vi "Menu Handler.vi"(8 "error in (no error)":errorcluster, 9 "ItemTag":string, 10 "Menu in":refnum<k9>, 11 "queue in":refnum<queue>) -> (0 "Error Out":errorcluster, 3 "Log 10?":bool=TRUE)   [LabVIEW 2014]
uses:
  Type Defs/OCT Hardware States.ctl
  DAQ Status States.ctl
  Classes/DAQ Control Functional Global States.ctl
  Classes/Processing/View A-Scan.vi
  Classes/Processing.lvclass
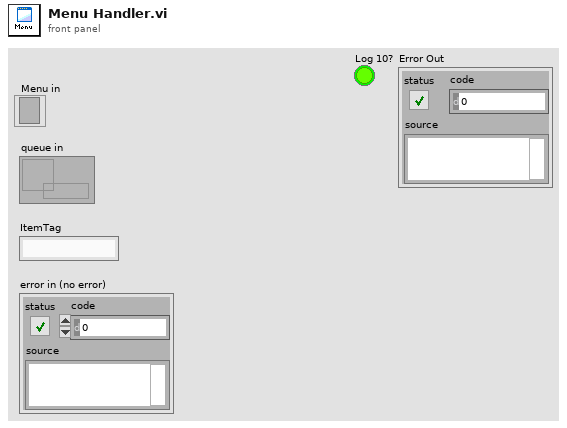
[diagram p1: front panel]
types:
  T1 = enum32{"Invalid", "Standard", "Closed", "Hidden", "Minimized", "Maximized"}
  T2 = typedef "DAQ Status States.ctl" = enum16{"Get", "Show"}
  T3 = typedef "OCT Hardware States.ctl" = enum16{"Acquire Data", "Initialize Laser", "Initialize Galvos", "Startup", "Reset DAQ", "Background Subtraction", "Acquire Background", "Update DAQ Parameters", "Stop", "Set Clock", "Initialize DAQ", "Set Resampling Array", "Save Sweep", "Configure Laser", "128 x 128", "512 x 1", "512 x 512", "Review Data"}
  T4 = typedef "DAQ Control Functional Global States.ctl" = enum16{"Status", "Set Processing Finished", "Reset", "Clear", "Set DAQ Finished"}
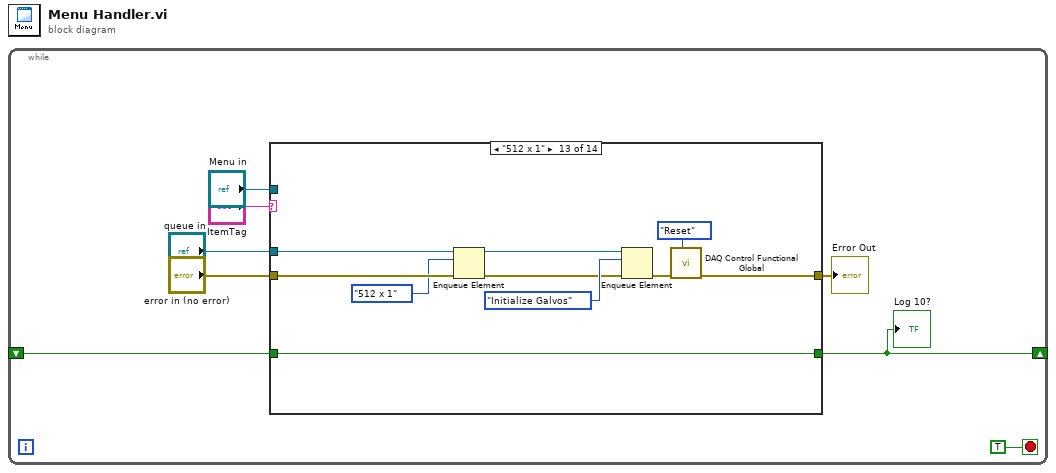
[diagram p0: block diagram]
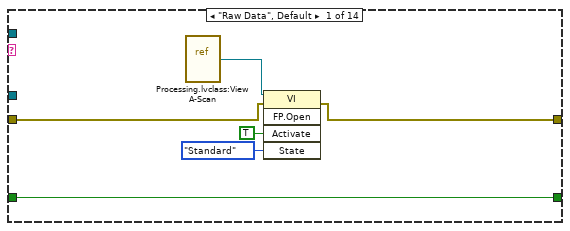
[diagram p2: hidden frame]
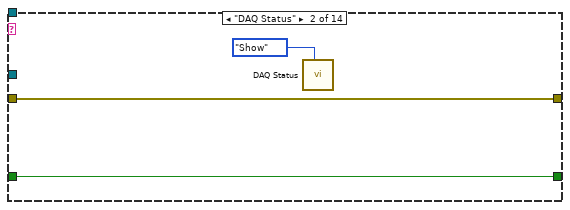
[diagram p3: hidden frame]
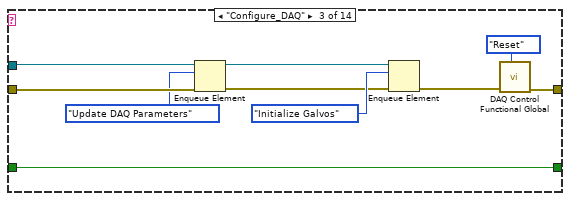
[diagram p4: hidden frame]
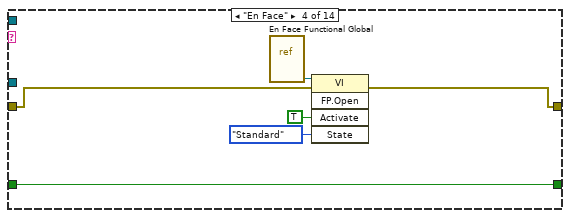
[diagram p5: hidden frame]
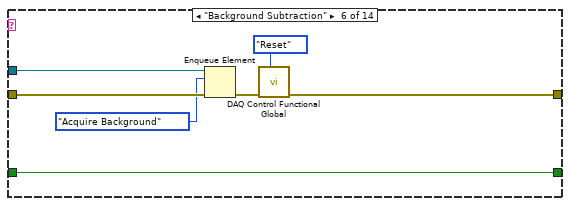
[diagram p7: hidden frame]
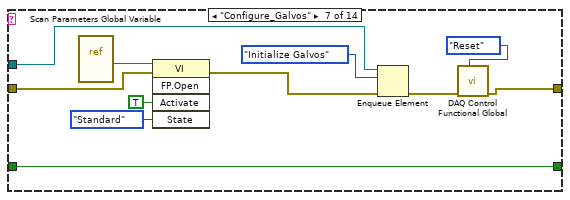
[diagram p8: hidden frame]
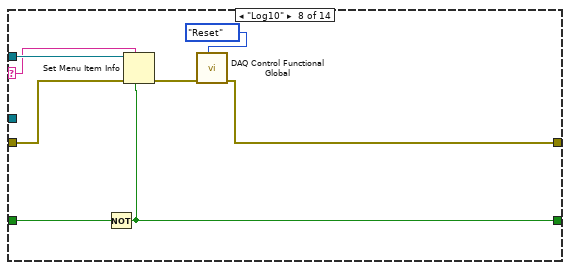
[diagram p9: hidden frame]
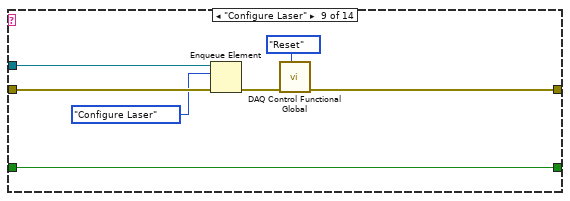
[diagram p10: hidden frame]
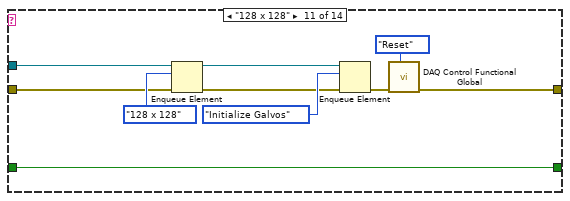
[diagram p12: hidden frame]
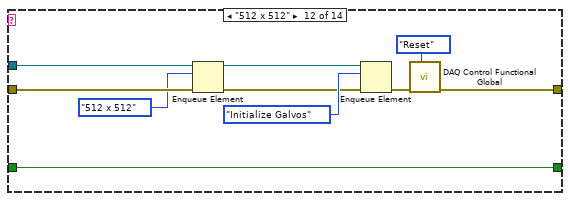
[diagram p13: hidden frame]
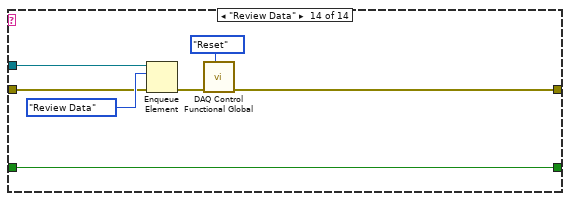
[diagram p14: hidden frame]
diagram:
  n1 = while {
    shift-right: [w2] -> _
    shift-left: _ -> [w3]
    stop <- TRUE stop-if-true
    n2 = case shown="\"512 x 1\"" "ItemTag" {
      selector: "ItemTag" -> [_ _ _ _ _ _ _ w60 _ _ _ _ _ _]
      tunnel: "queue in" -> [_ _ w27 _ _ w40 w47 _ w68 _ w74 w85 w95 w105]
      tunnel: "error in (no error)" -> [w9 w15 w26 w30 w34 w41 w45 w58 w67 w69 w73 w84 w94 w104]
      tunnel: "Menu in" -> [_ _ _ _ _ _ _ w61 _ _ _ _ _ _]
      tunnel: [w11 w16 w19 w29 w35 w37 w44 w55 w63 w70 w72 w82 w92 w102] -> w2
      tunnel: w3 -> [w11 w16 w19 w29 w35 w37 w44 w56 w63 w70 w72 w82 w92 w102]
      tunnel: [w10 w15 w18 w28 w34 w36 w43 w54 w62 w69 w71 w81 w91 w101] -> w1
      frame "Raw Data", Default {
        n3 = vi-ref "Processing.lvclass:View A-Scan.vi"() -> (w14:refnum<vi>)
        n4 = invoke class="VI" method="FP.Open"(reference=w14, error in=w9, "Activate"=TRUE ("Activate?"), "State"=T1."Standard") -> (error out=w10:errorcluster)  [unwired: 1 in, 4 out]
      }
      frame "DAQ Status" {
        n5 = call "DAQ Status.vi"("Enum"=DAQ_Status_States."Show") -> ()  [unwired: 9 in, 2 out]
      }
      frame "Configure_DAQ" {
        n6 = Enqueue Element(queue=w27, element=OCT_Hardware_States."Update DAQ Parameters", error in (no error)=w26) -> (queue out=w21:refnum<queue>, error out=w22:errorcluster)  [unwired: 1 in, 1 out]
        n7 = Enqueue Element(queue=w21, element=OCT_Hardware_States."Initialize Galvos", error in (no error)=w22) -> (error out=w20:errorcluster)  [unwired: 1 in, 2 out]
        n8 = call "DAQ Control Functional Global.vi"("State"=DAQ_Control_Functional_Global_States."Reset", "Error In"=w20) -> ("Error Out"=w18:errorcluster)  [unwired: 6 in, 3 out]
      }
      frame "En Face" {
        n9 = vi-ref "En Face Functional Global.vi"() -> (w31:refnum<vi>)
        n10 = invoke class="VI" method="FP.Open"(reference=w31, error in=w30, "Activate"=TRUE ("Activate?"), "State"=T1."Standard") -> (error out=w28:errorcluster)  [unwired: 1 in, 4 out]
      }
      frame "K-Space Correction" {
      }
      frame "Background Subtraction" {
        n11 = Enqueue Element(queue=w40, element=OCT_Hardware_States."Acquire Background", error in (no error)=w41) -> (error out=w38:errorcluster)  [unwired: 1 in, 2 out]
        n12 = call "DAQ Control Functional Global.vi"("State"=DAQ_Control_Functional_Global_States."Reset", "Error In"=w38) -> ("Error Out"=w36:errorcluster)  [unwired: 6 in, 3 out]
      }
      frame "Configure_Galvos" {
        n13 = vi-ref "Scan Parameters Global Variable.vi"() -> (w53:refnum<vi>)
        n14 = invoke class="VI" method="FP.Open"(reference=w53, error in=w45, "Activate"=TRUE ("Activate?"), "State"=T1."Standard") -> (error out=w46:errorcluster)  [unwired: 1 in, 4 out]
        n15 = Enqueue Element(queue=w47, element=OCT_Hardware_States."Initialize Galvos", error in (no error)=w46) -> (error out=w49:errorcluster)  [unwired: 1 in, 2 out]
        n16 = call "DAQ Control Functional Global.vi"("State"=DAQ_Control_Functional_Global_States."Reset", "Error In"=w49) -> ("Error Out"=w43:errorcluster)  [unwired: 6 in, 3 out]
      }
      frame "Log10" {
        n17 = Not(x=w56) -> (.not. x?=w55:bool)
        n18 = Set Menu Item Info(6:w55, 7:w60, 8:w58, 11:w61) -> (0:w57:errorcluster)  [unwired: 3 in, 1 out]
        n19 = call "DAQ Control Functional Global.vi"("State"=DAQ_Control_Functional_Global_States."Reset", "Error In"=w57) -> ("Error Out"=w54:errorcluster)  [unwired: 6 in, 3 out]
      }
      frame "Configure Laser" {
        n20 = Enqueue Element(queue=w68, element=OCT_Hardware_States."Configure Laser", error in (no error)=w67) -> (error out=w64:errorcluster)  [unwired: 1 in, 2 out]
        n21 = call "DAQ Control Functional Global.vi"("State"=DAQ_Control_Functional_Global_States."Reset", "Error In"=w64) -> ("Error Out"=w62:errorcluster)  [unwired: 6 in, 3 out]
      }
      frame "Laser Status" {
      }
      frame "128 x 128" {
        n22 = Enqueue Element(queue=w74, element=OCT_Hardware_States."128 x 128", error in (no error)=w73) -> (queue out=w76:refnum<queue>, error out=w77:errorcluster)  [unwired: 1 in, 1 out]
        n23 = Enqueue Element(queue=w76, element=OCT_Hardware_States."Initialize Galvos", error in (no error)=w77) -> (error out=w75:errorcluster)  [unwired: 1 in, 2 out]
        n24 = call "DAQ Control Functional Global.vi"("State"=DAQ_Control_Functional_Global_States."Reset", "Error In"=w75) -> ("Error Out"=w71:errorcluster)  [unwired: 6 in, 3 out]
      }
      frame "512 x 512" {
        n25 = Enqueue Element(queue=w85, element=OCT_Hardware_States."512 x 512", error in (no error)=w84) -> (queue out=w87:refnum<queue>, error out=w88:errorcluster)  [unwired: 1 in, 1 out]
        n26 = Enqueue Element(queue=w87, element=OCT_Hardware_States."Initialize Galvos", error in (no error)=w88) -> (error out=w86:errorcluster)  [unwired: 1 in, 2 out]
        n27 = call "DAQ Control Functional Global.vi"("State"=DAQ_Control_Functional_Global_States."Reset", "Error In"=w86) -> ("Error Out"=w81:errorcluster)  [unwired: 6 in, 3 out]
      }
      frame "512 x 1" {
        n28 = Enqueue Element(queue=w95, element=OCT_Hardware_States."512 x 1", error in (no error)=w94) -> (queue out=w97:refnum<queue>, error out=w98:errorcluster)  [unwired: 1 in, 1 out]
        n29 = Enqueue Element(queue=w97, element=OCT_Hardware_States."Initialize Galvos", error in (no error)=w98) -> (error out=w96:errorcluster)  [unwired: 1 in, 2 out]
        n30 = call "DAQ Control Functional Global.vi"("State"=DAQ_Control_Functional_Global_States."Reset", "Error In"=w96) -> ("Error Out"=w91:errorcluster)  [unwired: 6 in, 3 out]
      }
      frame "Review Data" {
        n31 = Enqueue Element(queue=w105, element=OCT_Hardware_States."Review Data", error in (no error)=w104) -> (error out=w103:errorcluster)  [unwired: 1 in, 2 out]
        n32 = call "DAQ Control Functional Global.vi"("State"=DAQ_Control_Functional_Global_States."Reset", "Error In"=w103) -> ("Error Out"=w101:errorcluster)  [unwired: 6 in, 3 out]
      }
    }
    "Log 10?" <- w2
    "Error Out" <- w1
  }
